vi "Build_Method.vi"(0 "AB_DepPackedLibrary in":refnum<class "AB_DepPackedLibrary.lvclass">, 1 "AppFlags":u32 format="%.0x", 2 "versionIndependent":bool, 3 "Zip path":path, 4 "Shell Path":path, 5 "error in (no error)":errorcluster, 6 "eng_consolidatedTypeInfo":string, 7 "Options string":string, 10 "buildContext":refnum<vi>, 11 "source project path":path, 12 "PackedLib path":path, 13 "eng_LEIFBuildDataCookie":u32) -> (14 "AB_DepPackedLibrary out":refnum<class "AB_DepPackedLibrary.lvclass">, 19 "error out":errorcluster)   [LabVIEW 2020, in "AB_DepPackedLibrary.lvclass"]
uses:
  <vilib>/AppBuilder/AB_Classes/DepPackedLib/AB_DepPackedLibrary.lvclass
  <vilib>/AppBuilder/AB_Classes/DepPackedLib/AB_DepPackedLibrary.lvclass/AB_DepPackedLibrary.ctl
  <vilib>/AppBuilder/AB_Classes/PackedLib/AB_PackedLibrary.lvclass
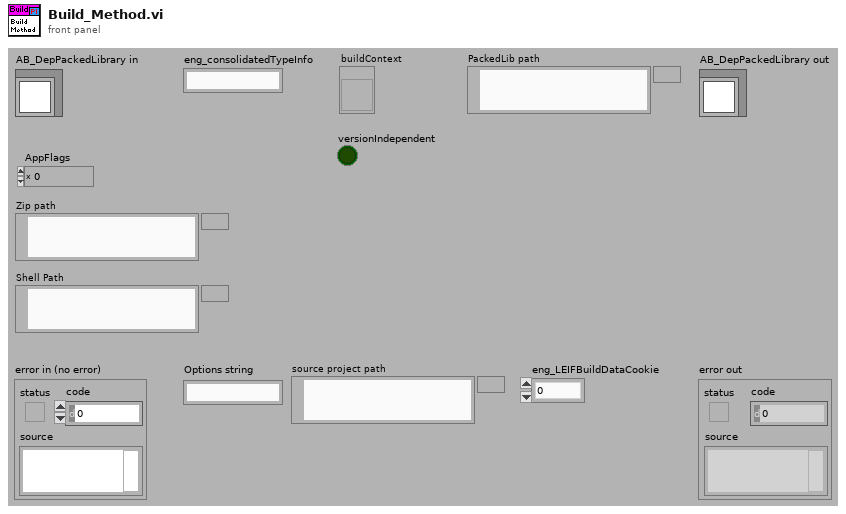
[diagram p1: front panel]
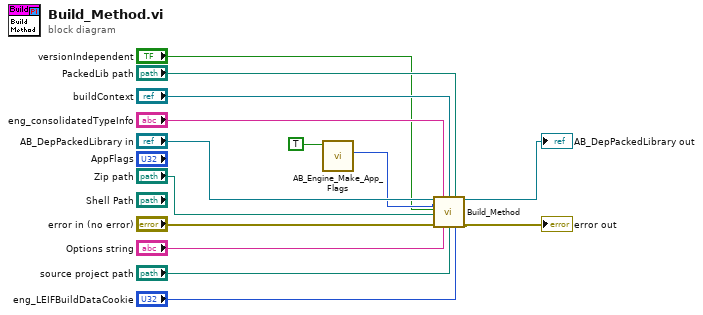
[diagram p0: block diagram]
diagram:
  n1 = call <vilib>:"AB_Engine_Make_App_Flags.vi"("LabVIEW RT?"=TRUE) -> ("AppFlags"=w7:u32)  [unwired: 3 in, 7 out]
  n2 = call-parent "Build_Method.vi"("AB_PackedLibrary in"="AB_DepPackedLibrary in", "AppFlags"=w7, "versionIndependent"="versionIndependent", "Zip path"="Zip path", "error in (no error)"="error in (no error)", "eng_consolidatedTypeInfo"="eng_consolidatedTypeInfo", "Options string"="Options string", "buildContext"="buildContext", "source project path"="source project path", "PackedLib path"="PackedLib path", "eng_LEIFBuildDataCookie"="eng_LEIFBuildDataCookie") -> ("AB_PackedLibrary out"=→"AB_DepPackedLibrary out":refnum<class "AB_DepPackedLibrary.lvclass">, "error out"=→"error out":errorcluster)  [unwired: 7 in]
